vi "test_next_steps_class_with_json_param.vi"(8 "error in (no error)":errorcluster) -> (0 "error out":errorcluster)   [LabVIEW 2023, in "Easy.SequenceManager.Test.lvlib"]
uses:
  Easy.SequenceManager.Test.lvlib
  src/SequenceManager/SequenceManager.lvclass
  src/Parameter/Parameter.lvclass
  src/Step/Step.lvclass
  <vilib>/addons/_JKI Toolkits/Caraya/classes/Test/Test.lvclass
  <vilib>/addons/_JKI Toolkits/Caraya/classes/Assert/Assert.lvclass
panel:
  out "Value":variant
  in  "SequenceManager in":refnum<class "SequenceManager.lvclass">
  # "Connector Pane"
  # "Locals"
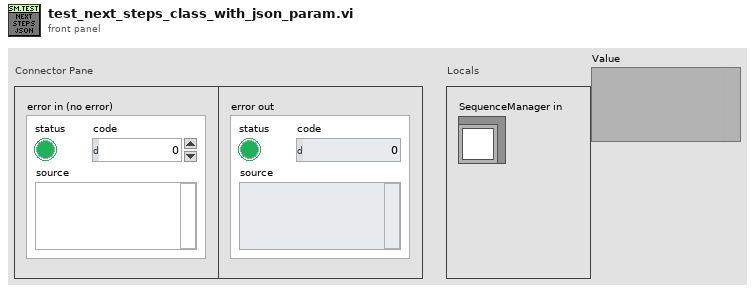
[diagram p1: front panel]
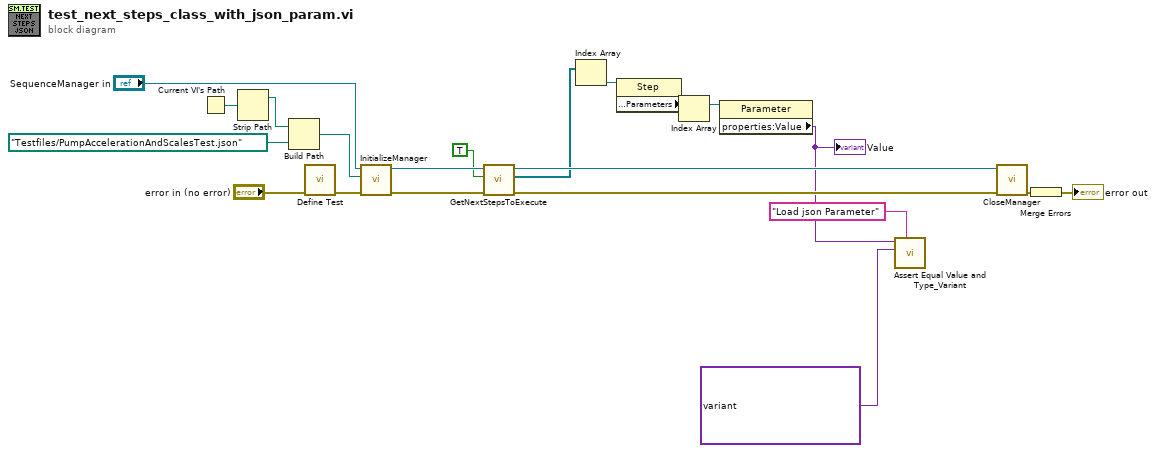
[diagram p0: block diagram]
diagram:
  n1 = Current VI's Path() -> (path=w20:path)
  n2 = Strip Path(path=w20) -> (stripped path=w14:path)  [unwired: 1 out]
  n3 = Build Path(base path=w14, name or relative path=path "Testfiles/PumpAccelerationAndScalesTest.json") -> (appended path=w15:path)
  n4 = call <vilib>:"Define Test.vi"("error in (no error)"="error in (no error)") -> ("error out"=w13:errorcluster)  [unwired: 9 in, 1 out]
  n5 = call-dynamic "InitializeManager.vi"("error in (no error)"=w13, "Path to JSON sequence file"=w15, "SequenceManager in"="SequenceManager in") -> ("error out"=w12:errorcluster, "SequenceManager out"=w16:refnum<class "SequenceManager.lvclass">)  [unwired: 7 in]
  n6 = call-dynamic "GetNextStepsToExecute.vi"("error in (no error)"=w12, "beautify JSON?"=TRUE, "SequenceManager in"=w16) -> ("error out"=w9:errorcluster, "Steps"=w7:refnum<class "Step.lvclass">[], "SequenceManager out"=w10:refnum<class "SequenceManager.lvclass">)  [unwired: 5 in, 1 out]
  n7 = Index Array(array=w7) -> (element=w6:refnum<class "Step.lvclass">)  [unwired: 1 in]
  n8 = property on="Property Node" class="Step"(reference=w6) -> ("properties:Parameters"=w5:refnum<class "Parameter.lvclass">[])  [unwired: 1 in, 2 out]
  n9 = Index Array(array=w5) -> (element=w4:refnum<class "Parameter.lvclass">)  [unwired: 1 in]
  n10 = property on="Property Node" class="Parameter"(reference=w4) -> ("properties:Value"=w3:variant)  [unwired: 1 in, 2 out]
  "Value" <- w3
  n11 = call <vilib>:"Assert Equal Value and Type_Variant.vi"("Label"="Load json Parameter", "Y"=variant(string "{\r\n          \"SampleRate\": 1000,\r\n          \"SamplesPerLoop\": 200\r\n        }") ("Value"), "X"=w3) -> ()  [unwired: 7 in, 2 out]
  n12 = call-dynamic "CloseManager.vi"("error in (no error)"=w9, "SequenceManager in"=w10) -> ("error out"=w11:errorcluster)  [unwired: 8 in, 1 out]
  n13 = Merge Errors(w11) -> (→"error out":errorcluster)
